vi "cmd_test.vi"() -> ()   [LabVIEW 2025]
panel:
  in  "Arguments":string
  out "String":string
  out "Std Error":dbl
  out "STD Out":string
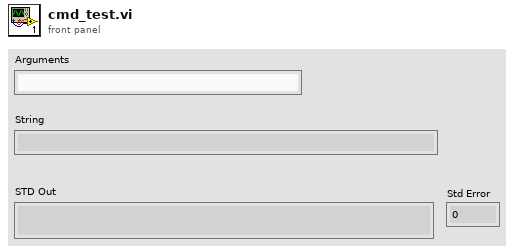
[diagram p1: front panel]
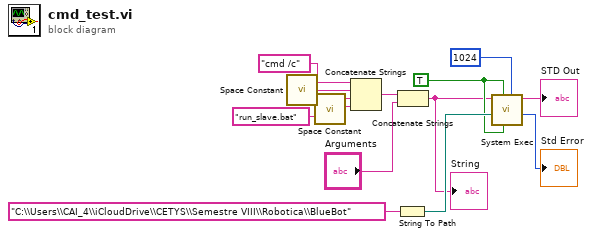
[diagram p0: block diagram]
diagram:
  w6 = TRUE
  n1 = call <vilib>:"Space Constant.vi"() -> ("String"=w11:string)
  n2 = call <vilib>:"Space Constant.vi"() -> ("String"=w4:string)
  n3 = Concatenate Strings("cmd /c", w11, "run_slave.bat", w4) -> (w3:string)
  n4 = String To Path(string="C:\\Users\\CAI_4\\iCloudDrive\\CETYS\\Semestre VIII\\Robotica\\BlueBot") -> (path=w9:path)
  n5 = Concatenate Strings(w3, "Arguments") -> (w2:string)
  "String" <- w2
  n6 = call <vilib>:"System Exec.vi"("expected output size  (4096)"=1024, "run minimized? (F)"=w6, "wait until completion? (T)"=w6, "working directory"=w9, "command line"=w2) -> ("return code"=→"Std Error":i32, "standard output"=→"STD Out":string)  [unwired: 3 in, 2 out]
